vi "Module Name--constant.vi"() -> (3 "Module Name":string)   [LabVIEW 2019, in "PowerElectronics0X45.lvlib"]
doc: "Return the name of the module that owns this VI. \n_____\nBased on DQMH Dev Tools: Project Template 7.1.0.1503."
uses:
  PowerElectronics0X45.lvlib
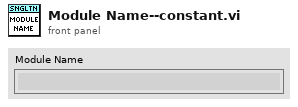
[diagram p1: front panel]
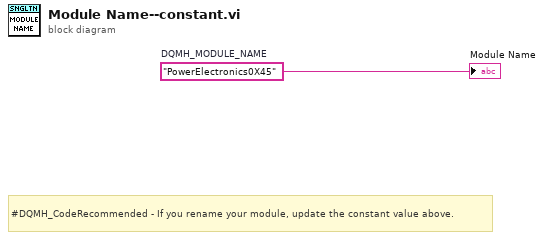
[diagram p0: block diagram]
diagram:
  w1 = "PowerElectronics0X45"  # DQMH_MODULE_NAME
  # "#DQMH_CodeRecommended - If you rename your module, update the constant value above."
  "Module Name" <- w1
